vi "Actor Core.vi"(8 "error in":errorcluster, 11 "AirMar150WX in":refnum<class "AirMar150WX.lvclass">) -> (0 "error out":errorcluster, 3 "Actor out":refnum<class "Actor.lvclass">)   [LabVIEW 2017, in "AirMar 150WX.lvlib" / "AirMar150WX.lvclass"]
doc: "(<B>Filename</B>: Actor Framework.lvlib:Actor.lvclass:Actor Core.vi)\n\nReceives messages to the actor, reacts to them, and initiates any error handling that may shut the actor down.\n\nDescendant classes may override this VI to append parallel tasks for the actor to complete while it handles messages. Overrides use the Call Parent Method node."
uses:
  AirMar150WX.lvclass
  C:/Program Files (x86)/National Instruments/LabVIEW 2017/vi.lib/ActorFramework/Actor/Actor.lvclass
  <vilib>/ActorFramework/Actor/Actor.lvclass
  <vilib>/ActorFramework/Actor/Actor.lvclass/Actor.ctl
  <vilib>/ActorFramework/Message Enqueuer/Message Enqueuer.lvclass/Message Enqueuer.ctl
  AirMar150WX.lvclass/AirMar150WX.ctl
  <vilib>/ActorFramework/Message Enqueuer/Init from Existing Queue.vi
  <vilib>/ActorFramework/Message Enqueuer/Enqueue.vi
  <vilib>/ActorFramework/Stop Msg/Stop Msg.lvclass
  C:/Program Files (x86)/National Instruments/LabVIEW 2017/vi.lib/ActorFramework/Message/Message.lvclass
  <vilib>/ActorFramework/Message Priority Queue/Priority Enqueue.vi
  Sensor Actor/Sensor/Sensor.lvclass
  <vilib>/ActorFramework/Message Enqueuer/Message Enqueuer.lvclass
  AirMar150WX Messages/Measure AirMar150WX Msg/Measure AirMar150WX Msg.lvclass
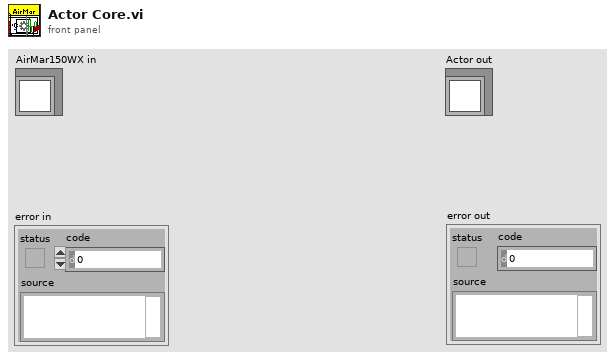
[diagram p1: front panel]
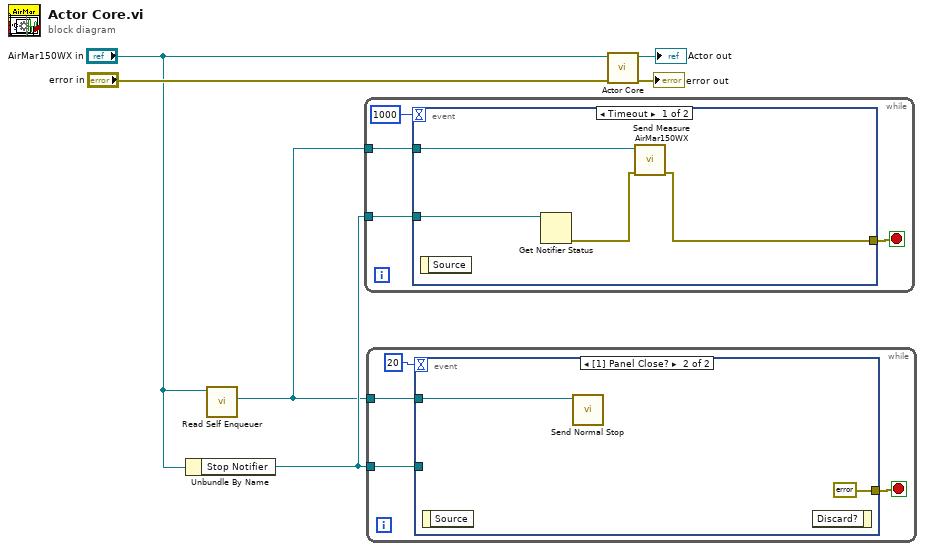
[diagram p0: block diagram]
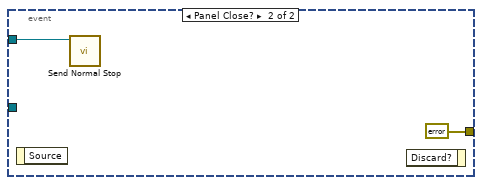
[diagram p2: hidden frame]
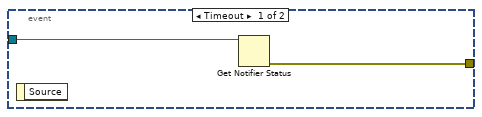
[diagram p3: hidden frame]
diagram:
  n1 = Unbundle By Name("AirMar150WX in") -> ("Stop Notifier"=w2:refnum<notifier>)
  n2 = call <vilib>:"Read Self Enqueuer.vi"("Actor"="AirMar150WX in") -> ("Self Enqueuer"=w1:refnum<class "Message Enqueuer.lvclass">)  [unwired: 10 in]
  n3 = while {
    tunnel: w1 -> [w9]
    tunnel: w2 -> [w10]
    stop <- w7 stop-if-true
    n4 = event shown="[0] Timeout" {
      selector: _ -> [_ _]
      dyn-events: _ -> [_ _]
      timeout: 1000 -> [_ _]
      tunnel: w10 -> [w14 _]
      tunnel: w9 -> [w13 w16]
      tunnel: [w11 errorcluster {"status"=TRUE, "code"=0, "source"=""} ("error out")] -> w7
      event Timeout {
        n5 = event-data() -> ()  [unwired: 1 in, 1 out]
        n6 = Get Notifier Status(notifier=w14) -> (error out=w12:errorcluster)  [unwired: 1 in, 4 out]
        n7 = call "Send Measure AirMar150WX.vi"("error in (no error)"=w12, "Message Enqueuer in"=w13) -> ("error out"=w11:errorcluster)  [unwired: 8 in, 1 out]
      }
      event Panel Close? {
        n8 = event-data() -> ()  [unwired: 1 in, 1 out]
        n9 = call <vilib>:"Send Normal Stop.vi"("Message Enqueuer"=w16) -> ()  [unwired: 10 in, 1 out]
        n10 = event-data() -> ()  [unwired: 2 in, 1 out]
      }
    }
  }
  n11 = while {
    tunnel: w1 -> [w19]
    tunnel: w2 -> [w20]
    stop <- w17 stop-if-true
    n12 = event shown="[1] Panel Close?" {
      selector: _ -> [_ _]
      dyn-events: _ -> [_ _]
      timeout: 20 -> [_ _]
      tunnel: w20 -> [w22 _]
      tunnel: w19 -> [_ w24]
      tunnel: [w21 errorcluster {"status"=TRUE, "code"=0, "source"=""} ("error out")] -> w17
      event Timeout {
        n13 = event-data() -> ()  [unwired: 1 in, 1 out]
        n14 = Get Notifier Status(notifier=w22) -> (error out=w21:errorcluster)  [unwired: 1 in, 4 out]
      }
      event Panel Close? {
        n15 = event-data() -> ()  [unwired: 1 in, 1 out]
        n16 = call <vilib>:"Send Normal Stop.vi"("Message Enqueuer"=w24) -> ()  [unwired: 10 in, 1 out]
        n17 = event-data() -> ()  [unwired: 2 in, 1 out]
      }
    }
  }
  n18 = call-parent "Actor Core.vi"("error in"="error in", "Sensor in"="AirMar150WX in") -> ("error out"=→"error out":errorcluster, "Actor out"=→"Actor out":refnum<class "Actor.lvclass">)  [unwired: 8 in]
